vi "mindsensors devices.vi"   [LabVIEW 2010]
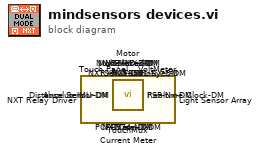
[diagram p0: block diagram]
diagram:
  n1 = call <vilib>:"TouchMux.vi"() -> ()  [unwired: 3 in, 2 out]
  n2 = call "Touch Panel.vi"() -> ()  [unwired: 3 in, 2 out]
  n3 = call <vilib>:"NXT Relay Driver.vi"() -> ()  [unwired: 4 in, 1 out]
  n4 = call <vilib>:"Light Sensor Array.vi"() -> ()  [unwired: 3 in, 2 out]
  n5 = call <vilib>:"Current Meter.vi"() -> ()  [unwired: 3 in, 2 out]
  n6 = call <vilib>:"VoltMeter.vi"() -> ()  [unwired: 3 in, 2 out]
  n7 = call <vilib>:"NumericPad-DM.vi"() -> ()  [unwired: 3 in, 2 out]
  n8 = call <vilib>:"NXTMMX-DM.vi"() -> ()  [unwired: 3 in, 2 out]
  n9 = call <vilib>:"PCF8574-NX-DM.vi"() -> ()  [unwired: 3 in, 2 out]
  n10 = call <vilib>:"PCF8591-NX-DM.vi"() -> ()  [unwired: 3 in, 2 out]
  n11 = call <vilib>:"Motor Multiplexer-DM.vi"() -> ()  [unwired: 3 in, 2 out]
  n12 = call <vilib>:"RXMux-DM.vi"() -> ()  [unwired: 3 in, 2 out]
  n13 = call <vilib>:"NXTCam-DM.vi"() -> ()  [unwired: 3 in, 2 out]
  n14 = call <vilib>:"AbsoluteIMU-DM.vi"() -> ()  [unwired: 3 in, 2 out]
  n15 = call <vilib>:"Realtime Clock-DM.vi"() -> ()  [unwired: 3 in, 2 out]
  n16 = call <vilib>:"NXTServo-DM.vi"() -> ()  [unwired: 3 in, 2 out]
  n17 = call <vilib>:"NXTHID-DM.vi"() -> ()  [unwired: 3 in, 2 out]
  n18 = call <vilib>:"PFMate-DM.vi"() -> ()  [unwired: 4 in, 1 out]
  n19 = call <vilib>:"Distance Sensor-DM.vi"() -> ()  [unwired: 3 in, 2 out]
  n20 = call <vilib>:"PSP-Nx-DM.vi"() -> ()  [unwired: 3 in, 2 out]
  n21 = call <vilib>:"NXTSumoEyes-DM.vi"() -> ()  [unwired: 3 in, 2 out]
